vi "Get TagDistance By Tag ID.vi"(9 "TagDistanceArray":T1(array[cluster]), 10 "TagID":dbl) -> (2 "Distance":dbl)   [LabVIEW 2014, in "Anchor.lvclass"]
uses:
  Anchor.lvclass
  Tag.lvclass
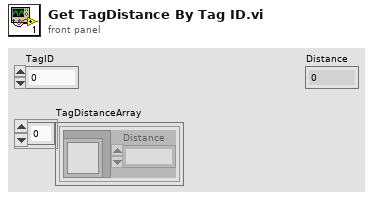
[diagram p1: front panel]
types:
  T1 = cluster{"Tag.lvclass":refnum<class "Tag.lvclass">, "Distance":dbl}[]
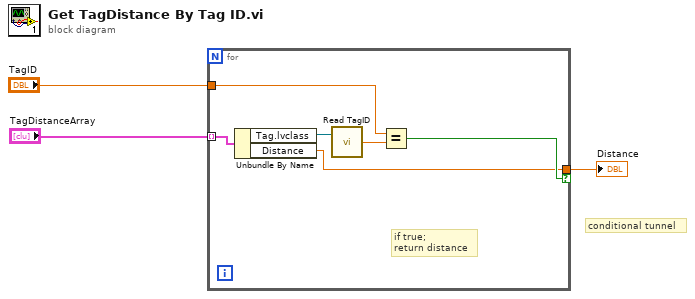
[diagram p0: block diagram]
diagram:
  # "conditional tunnel"
  n1 = for {
    tunnel: "TagDistanceArray" -> [w9] mode=indexing
    tunnel: "TagID" -> [w7]
    tunnel: [w4] -> w1 if=w5
    # "if true;\nreturn distance"
    n2 = Unbundle By Name(w9) -> ("Tag.lvclass"=w8:refnum<class "Tag.lvclass">, "Distance"=w4:dbl)
    n3 = call-dynamic "Read TagID.vi"("Tag in"=w8) -> ("TagID"=w6:dbl)  [unwired: 1 in, 2 out]
    n4 = Equal?(x=w7, y=w6) -> (x = y?=w5:bool)
  }
  "Distance" <- w1
